vi "Overzicht axes.vi"() -> (1 "Data out":T2(array[cluster])=[{"Name"="XLS_312", "Data"="XLS1=312", "Enum type"=enum."XLS with 312 nm resolution"}, {"Name"="XLS_1250", "Data"="XLS1=1250", "Enum type"=enum."XLS with 1250 nm resolution"}, {"Name"="XLS_78", "Data"="XLS1=78", "Enum type"=enum."XLS with 78nm resolution"}, {"Name"="XLS_5", "Data"="XLS1=5", "Enum type"=enum."XLS with 5nm resolution"}, {"Name"="XLS_1", "Data"="XLS1=1", "Enum type"=enum."XLS with 1 nm resolution"}, {"Name"="XLS_312_3N", "Data"="XLS3=312", "Enum type"=enum."XLS with 312 nm resolution"}, {"Name"="XLS_1250_3N", "Data"="XLS3=1250", "Enum type"=enum."XLS with 1250 nm resolution"}, {"Name"="XLS_78_3N", "Data"="XLS3=78", "Enum type"=enum."XLS with 78nm resolution"}, {"Name"="XLS_5_3N", "Data"="XLS3=5", "Enum type"=enum."XLS with 5nm resolution"}, {"Name"="XLS_1_3N", "Data"="XLS3=1", "Enum type"=enum."XLS with 1 nm resolution"}, {"Name"="XLA_312", "Data"="XLA1=312", "Enum type"=enum."XLA with 312 nm resolution"}, {"Name"="XLA_1250", "Data"="XLA1=1250", "Enum type"=enum."XLA with 1250 nm resolution"}, {"Name"="XLA_78", "Data"="XLA1=78", "Enum type"=enum."XLA with 78 nm resolution"}, {"Name"="XLA_312_3N", "Data"="XLA3=312", "Enum type"=enum."XLA with 312 nm resolution"}, {"Name"="XLA_1250_3N", "Data"="XLA3=1250", "Enum type"=enum."XLA with 1250 nm resolution"}, {"Name"="XLA_78_3N", "Data"="XLA3=78", "Enum type"=enum."XLA with 78 nm resolution"}, {"Name"="XLA_312_5N", "Data"="XLA3=312", "Enum type"=enum."XLA with 312 nm resolution"}, {"Name"="XLA_1250_5N", "Data"="XLA3=1250", "Enum type"=enum."XLA with 1250 nm resolution"}, {"Name"="XLA_78_5N", "Data"="XLA3=78", "Enum type"=enum."XLA with 78 nm resolution"}, {"Name"="XLA_312_10N", "Data"="XLA3=312", "Enum type"=enum."XLA with 312 nm resolution"}, {"Name"="XLA_1250_10N", "Data"="XLA3=1250", "Enum type"=enum."XLA with 1250 nm resolution"}, {"Name"="XLA_78_10N", "Data"="XLA3=78", "Enum type"=enum."XLA with 78 nm resolution"}, {"Name"="XRTA", "Data"="XRTA=109", "Enum type"=enum."XRT-A with 109 µrad resolution"}, {"Name"="XRTU_40_3", "Data"="XRT1=2", "Enum type"=enum."XRT-U-40 with 3 µrad resolution"}, {"Name"="XRTU_40_19", "Data"="XRT1=18", "Enum type"=enum."XRT-U-40 with 19 µrad resolution"}, {"Name"="XRTU_40_49", "Data"="XRT1=47", "Enum type"=enum."XRT-U 40 with 49 µrad resolution"}, {"Name"="XRTU_40_109", "Data"="XRT1=73", "Enum type"=enum."XRT-U-40 with 109 µrad resolution"}, {"Name"="XRTU_30_3", "Data"="XRT1=3", "Enum type"=enum."XRT-U-30 with 3 µrad resolution"}, {"Name"="XRTU_30_19", "Data"="XRT1=19", "Enum type"=enum."XRT-U-30 with 19 µrad resolution"}, {"Name"="XRTU_30_49", "Data"="XRT1=49", "Enum type"=enum."XRT-U-30 with 49 µrad resolution"}, {"Name"="XRTU_30_109", "Data"="XRT1=109", "Enum type"=enum."XRT-U-30 with 109 µrad resolution"}, {"Name"="XRTU_60_3", "Data"="XRT3=3", "Enum type"=enum."XRT-U-60 with 3 µrad resolution"}, {"Name"="XRTU_60_19", "Data"="XRT3=19", "Enum type"=enum."XRT-U-60 with 19 µrad resolution"}, {"Name"="XRTU_60_49", "Data"="XRT3=49", "Enum type"=enum."XRT-U-60 with 49 µrad resolution"}, {"Name"="XRTU_60_109", "Data"="XRT3=109", "Enum type"=enum."XRT-U-60 with 109 µrad resolution"}])   [LabVIEW 2019]
uses:
  Axis enum.ctl
panel:
  in  "Data":T2(array[cluster])=[{"Name"="XLS_312", "Data"="XLS1=312", "Enum type"=enum."XLS with 312 nm resolution"}, {"Name"="XLS_1250", "Data"="XLS1=1250", "Enum type"=enum."XLS with 1250 nm resolution"}, {"Name"="XLS_78", "Data"="XLS1=78", "Enum type"=enum."XLS with 78nm resolution"}, {"Name"="XLS_5", "Data"="XLS1=5", "Enum type"=enum."XLS with 5nm resolution"}, {"Name"="XLS_1", "Data"="XLS1=1", "Enum type"=enum."XLS with 1 nm resolution"}, {"Name"="XLS_312_3N", "Data"="XLS3=312", "Enum type"=enum."XLS with 312 nm resolution"}, {"Name"="XLS_1250_3N", "Data"="XLS3=1250", "Enum type"=enum."XLS with 1250 nm resolution"}, {"Name"="XLS_78_3N", "Data"="XLS3=78", "Enum type"=enum."XLS with 78nm resolution"}, {"Name"="XLS_5_3N", "Data"="XLS3=5", "Enum type"=enum."XLS with 5nm resolution"}, {"Name"="XLS_1_3N", "Data"="XLS3=1", "Enum type"=enum."XLS with 1 nm resolution"}, {"Name"="XLA_312", "Data"="XLA1=312", "Enum type"=enum."XLA with 312 nm resolution"}, {"Name"="XLA_1250", "Data"="XLA1=1250", "Enum type"=enum."XLA with 1250 nm resolution"}, {"Name"="XLA_78", "Data"="XLA1=78", "Enum type"=enum."XLA with 78 nm resolution"}, {"Name"="XLA_312_3N", "Data"="XLA3=312", "Enum type"=enum."XLA with 312 nm resolution"}, {"Name"="XLA_1250_3N", "Data"="XLA3=1250", "Enum type"=enum."XLA with 1250 nm resolution"}, {"Name"="XLA_78_3N", "Data"="XLA3=78", "Enum type"=enum."XLA with 78 nm resolution"}, {"Name"="XLA_312_5N", "Data"="XLA3=312", "Enum type"=enum."XLA with 312 nm resolution"}, {"Name"="XLA_1250_5N", "Data"="XLA3=1250", "Enum type"=enum."XLA with 1250 nm resolution"}, {"Name"="XLA_78_5N", "Data"="XLA3=78", "Enum type"=enum."XLA with 78 nm resolution"}, {"Name"="XLA_312_10N", "Data"="XLA3=312", "Enum type"=enum."XLA with 312 nm resolution"}, {"Name"="XLA_1250_10N", "Data"="XLA3=1250", "Enum type"=enum."XLA with 1250 nm resolution"}, {"Name"="XLA_78_10N", "Data"="XLA3=78", "Enum type"=enum."XLA with 78 nm resolution"}, {"Name"="XRTA", "Data"="XRTA=109", "Enum type"=enum."XRT-A with 109 µrad resolution"}, {"Name"="XRTU_40_3", "Data"="XRT1=2", "Enum type"=enum."XRT-U-40 with 3 µrad resolution"}, {"Name"="XRTU_40_19", "Data"="XRT1=18", "Enum type"=enum."XRT-U-40 with 19 µrad resolution"}, {"Name"="XRTU_40_49", "Data"="XRT1=47", "Enum type"=enum."XRT-U 40 with 49 µrad resolution"}, {"Name"="XRTU_40_109", "Data"="XRT1=73", "Enum type"=enum."XRT-U-40 with 109 µrad resolution"}, {"Name"="XRTU_30_3", "Data"="XRT1=3", "Enum type"=enum."XRT-U-30 with 3 µrad resolution"}, {"Name"="XRTU_30_19", "Data"="XRT1=19", "Enum type"=enum."XRT-U-30 with 19 µrad resolution"}, {"Name"="XRTU_30_49", "Data"="XRT1=49", "Enum type"=enum."XRT-U-30 with 49 µrad resolution"}, {"Name"="XRTU_30_109", "Data"="XRT1=109", "Enum type"=enum."XRT-U-30 with 109 µrad resolution"}, {"Name"="XRTU_60_3", "Data"="XRT3=3", "Enum type"=enum."XRT-U-60 with 3 µrad resolution"}, {"Name"="XRTU_60_19", "Data"="XRT3=19", "Enum type"=enum."XRT-U-60 with 19 µrad resolution"}, {"Name"="XRTU_60_49", "Data"="XRT3=49", "Enum type"=enum."XRT-U-60 with 49 µrad resolution"}, {"Name"="XRTU_60_109", "Data"="XRT3=109", "Enum type"=enum."XRT-U-60 with 109 µrad resolution"}]
  in  "Tabel":string[][](array[string])=[["XLS_312", "True", "XLS1=312", "312.5", "1000"], ["XLS_1250", "True", "XLS1=1250", "1250", "1000"], ["XLS_78", "True", "XLS1=78", "78.125", "1000"], ["XLS_5", "True", "XLS1=5", "5", "1000"], ["XLS_1", "True", "XLS1=1", "1", "1000"], ["XLS_312_3N", "True", "XLS3=312", "312.5", "1000"], ["XLS_1250_3N", "True", "XLS3=1250", "1250", "1000"], ["XLS_78_3N", "True", "XLS3=78", "78.125", "1000"], ["XLS_5_3N", "True", "XLS3=5", "5", "1000"], ["XLS_1_3N", "True", "XLS3=1", "1", "1000"], ["XLA_312", "True", "XLA1=312", "312.5", "1000"], ["XLA_1250", "True", "XLA1=1250", "1250", "1000"], ["XLA_78", "True", "XLA1=78", "78.125", "1000"], ["XLA_312_3N", "True", "XLA3=312", "312.5", "1000"], ["XLA_1250_3N", "True", "XLA3=1250", "1250", "1000"], ["XLA_78_3N", "True", "XLA3=78", "78.125", "1000"], ["XLA_312_5N", "True", "XLA3=312", "312.5", "1000"], ["XLA_1250_5N", "True", "XLA3=1250", "1250", "1000"], ["XLA_78_5N", "True", "XLA3=78", "78.125", "1000"], ["XLA_312_10N", "True", "XLA3=312", "312.5", "1000"], ["XLA_1250_10N", "True", "XLA3=1250", "1250", "1000"], ["XLA_78_10N", "True", "XLA3=78", "78.125", "1000"], ["XRTA", "False", "XRTA=109", "2*math.pi*1e6)/57600", "100"], ["XRTU_40_3", "False", "XRT1=2", "(2*math.pi*1e6)/2764800", "100"], ["XRTU_40_19", "False", "XRT1=18", "(2*math.pi*1e6)/345600", "100"], ["XRTU_40_49", "False", "XRT1=47", "(2*math.pi*1e6)/135000", "100"], ["XRTU_40_109", "False", "XRT1=73", "(2*math.pi*1e6)/86400", "100"], ["XRTU_30_3", "False", "XRT1=3", "(2*math.pi*1e6)/1843200", "100"], ["XRTU_30_19", "False", "XRT1=19", "(2*math.pi*1e6)/360000", "100"], ["XRTU_30_49", "False", "XRT1=49", "(2*math.pi*1e6)/144000", "100"], ["XRTU_30_109", "False", "XRT1=109", "(2*math.pi*1e6)/57600", "100"], ["XRTU_60_3", "False", "XRT3=3", "(2*math.pi*1e6)/2073600", "100"], ["XRTU_60_19", "False", "XRT3=19", "(2*math.pi*1e6)/324000", "100"], ["XRTU_60_49", "False", "XRT3=49", "(2*math.pi*1e6)/129600", "100"], ["XRTU_60_109", "False", "XRT3=109", "(2*math.pi*1e6)/64800", "100"], ["", "", "", "", ""]]
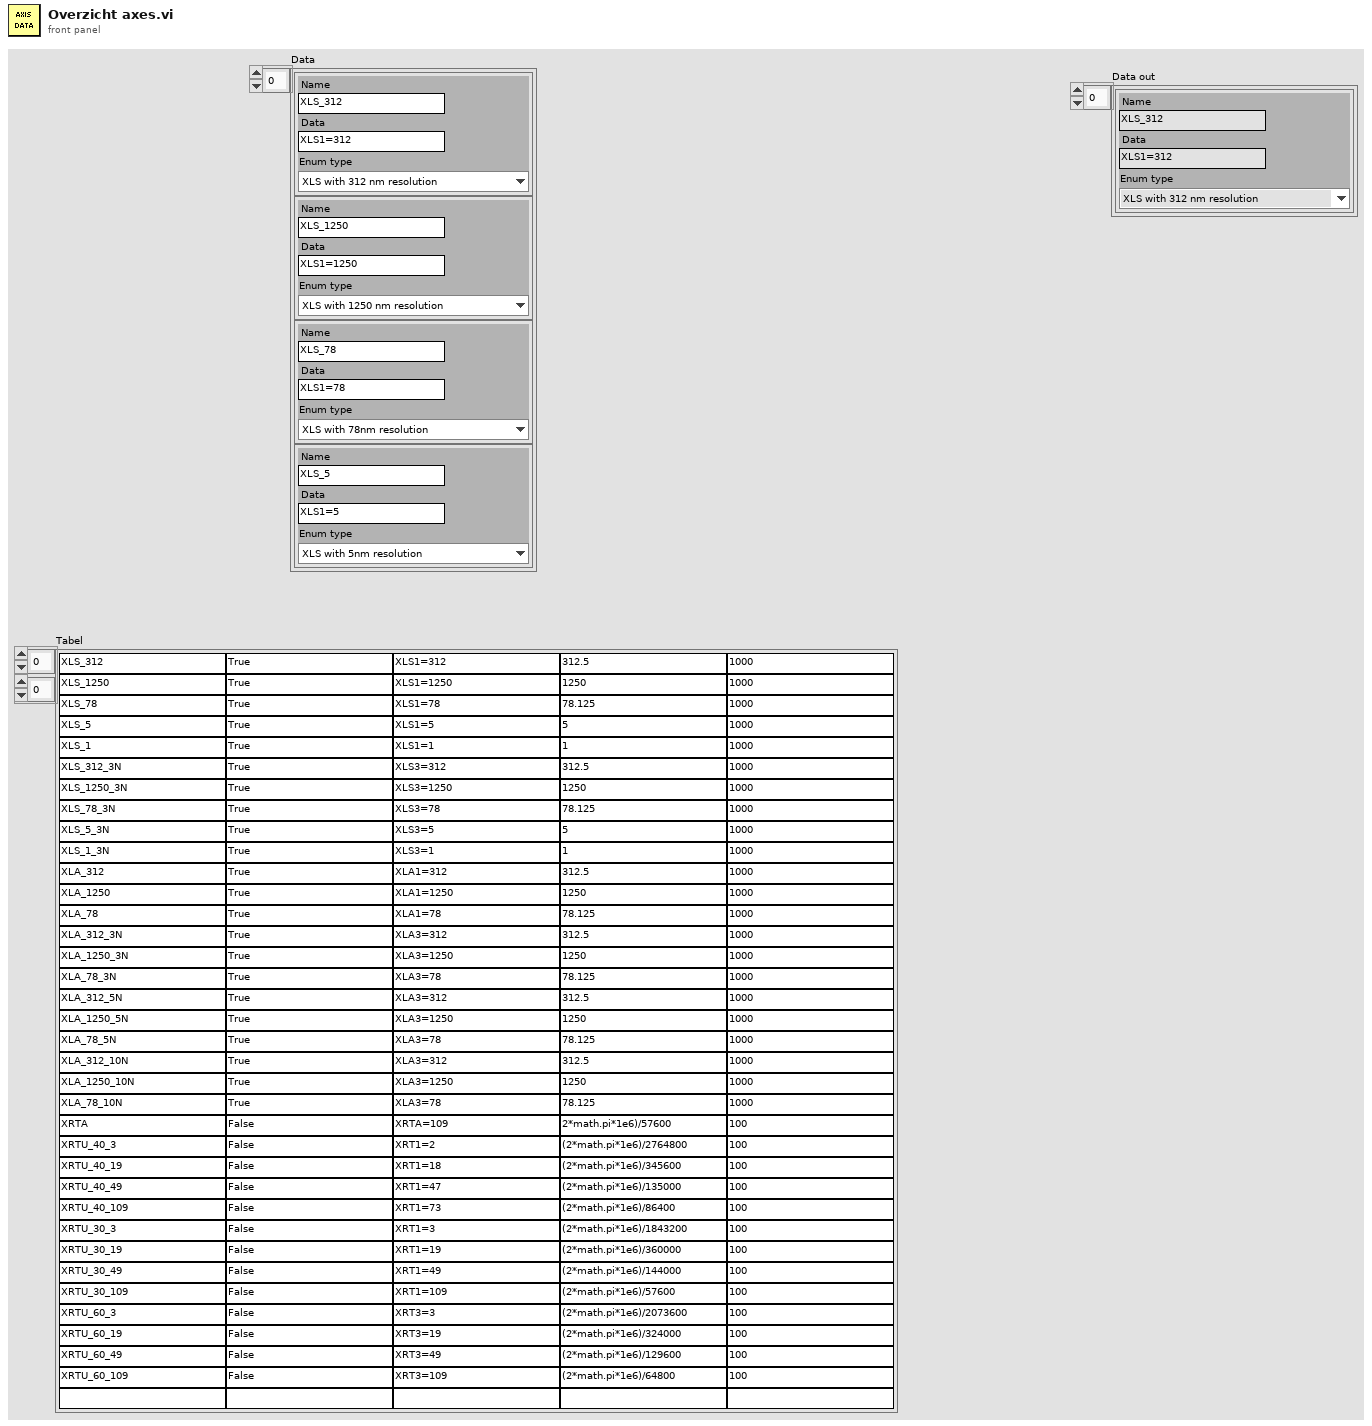
[diagram p1: front panel]
types:
  T1 = typedef "Axis enum.ctl" = enum16{"XLA with 50 µm resolution", "XLA with 10 µm resolution", "XLA with 1250 nm resolution", "XLA with 312 nm resolution", "XLA with 78 nm resolution", "XLS with 1250 nm resolution", "XLS with 312 nm resolution", "XLS with 78nm resolution", "XLS with 5nm resolution", "XLS with 1 nm resolution", "XRT-A with 109 µrad resolution", "XRT-U-30 with 109 µrad resolution", "XRT-U-30 with 49 µrad resolution", "XRT-U-30 with 19 µrad resolution", "XRT-U-30 with 3 µrad resolution", "XRT-U-40 with 109 µrad resolution", "XRT-U 40 with 49 µrad resolution", "XRT-U-40 with 19 µrad resolution", "XRT-U-40 with 3 µrad resolution", "XRT-U-60 with 109 µrad resolution", "XRT-U-60 with 49 µrad resolution", "XRT-U-60 with 19 µrad resolution", "XRT-U-60 with 3 µrad resolution"}
  T2 = cluster{"Name":string, "Data":string, "Enum type":T1}[]
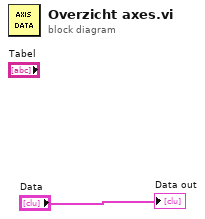
[diagram p0: block diagram]
diagram:
  "Data out" <- "Data"
